vi "DriveControl.vi"(5 "RobotDriveDevRef":T1={"DevStatus"={"status"=FALSE, "code"=0, "source"=""}, "Motors[]"=[], "Square Inputs"=FALSE, "Max Output"=1.0, "Isochronous"=FALSE}, 7 "Xvalue of Target":dbl, 8 "Right axis value":dbl, 9 "Left axis value":dbl, 10 "Lower Bound":dbl, 11 "Upper Bound":dbl) -> ()   [LabVIEW 2011]
uses:
  <vilib>/Rock Robotics/WPI/RobotDrive/WPI_RobotDriveDevRef.ctl
  <vilib>/Rock Robotics/WPI/MotorControl/WPI_MotorControlDeviceRef.ctl
  <vilib>/Rock Robotics/SystemInterfaces/Typedef/FPGA_TypedefDigitalModule.ctl
  <vilib>/Rock Robotics/SystemInterfaces/DIO/FPGA_DIOPWMChannel.ctl
  <vilib>/Rock Robotics/WPI/PWM/WPI_PWMDeadband.ctl
  <vilib>/Rock Robotics/WPI/CAN/Jaguar/SubVIs/WPI_CANJaguar_ControlMode.ctl
  <vilib>/Rock Robotics/WPI/PWM/WPI_PWMTransform_ConPane.ctl
panel:
  in  "Joystick value":dbl
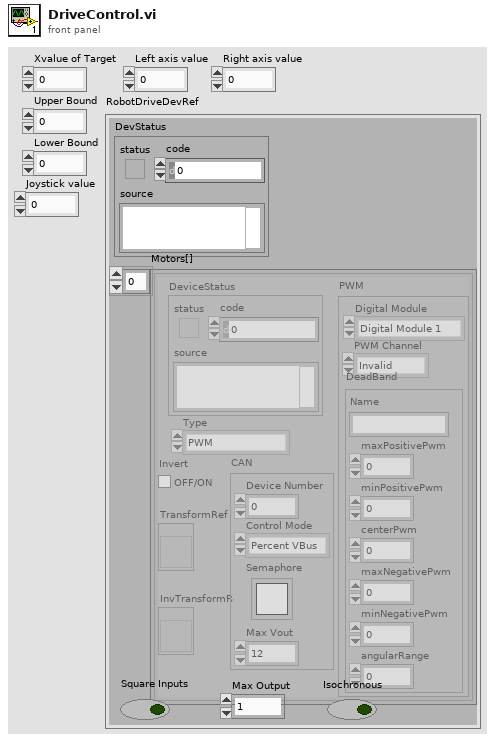
[diagram p1: front panel]
types:
  T1 = typedef "WPI_RobotDriveDevRef.ctl" = cluster{"DevStatus":errorcluster, "Motors[]":T2[], "Square Inputs":bool, "Max Output":dbl, "Isochronous":bool}
  T2 = typedef "WPI_MotorControlDeviceRef.ctl" = cluster{"DeviceStatus":errorcluster, "Type":enum16{"PWM", "CAN"}, "PWM":cluster{"Digital Module":T3, "PWM Channel":T4, "DeadBand":T5}, "CAN":cluster{"Device Number":u8, "Control Mode":T6, "Semaphore":T7, "Max Vout":dbl}, "Invert":bool, "TransformRef":T8, "InvTransformRef":T8}
  T3 = typedef "FPGA_TypedefDigitalModule.ctl" = enum16{"Digital Module 1", "Digital Module 2"}
  T4 = typedef "FPGA_DIOPWMChannel.ctl" = enum8{"PWM 1", "PWM 2", "PWM 3", "PWM 4", "PWM 5", "PWM 6", "PWM 7", "PWM 8", "PWM 9", "PWM 10", "Invalid"}
  T5 = typedef "WPI_PWMDeadband.ctl" = cluster{"Name":string, "maxPositivePwm":i32, "minPositivePwm":i32, "centerPwm":i32, "maxNegativePwm":i32, "minNegativePwm":i32, "angularRange":u16}
  T6 = typedef "WPI_CANJaguar_ControlMode.ctl" = enum8{"Percent VBus", "Current", "Speed", "Position", "Voltage"}
  T7 = typedef "Semaphore RefNum" = refnum<k1>
  T8 = typedef "WPI_PWMTransform_ConPane.ctl" = refnum<vi>
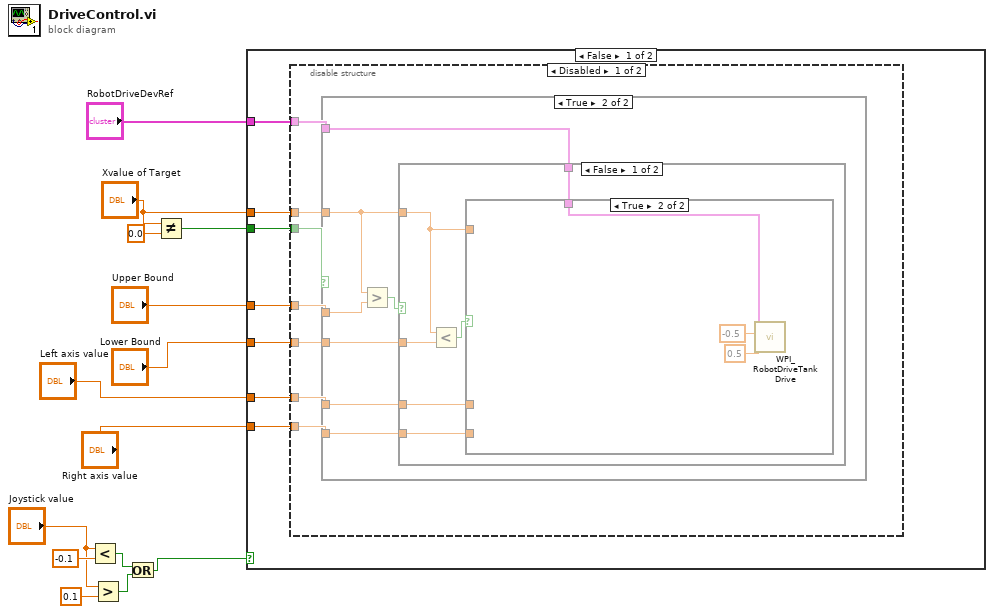
[diagram p0: block diagram]
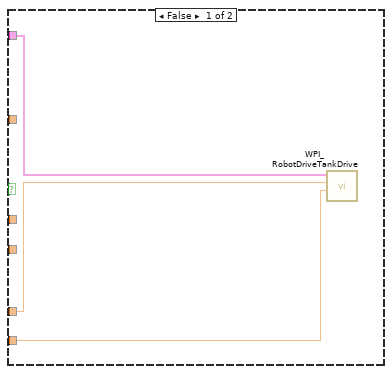
[diagram p2: hidden frame]
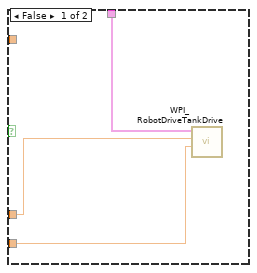
[diagram p3: hidden frame]
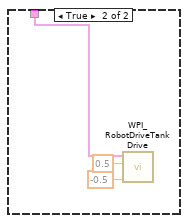
[diagram p4: hidden frame]
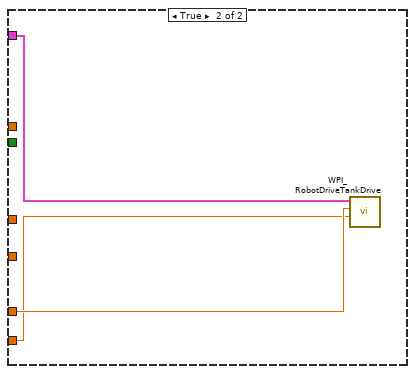
[diagram p6: hidden frame]
diagram:
  n1 = Less?(x="Joystick value", y=-0.1) -> (x < y?=w3:bool)
  n2 = Greater?(x="Joystick value", y=0.1) -> (0:w2:bool)
  n3 = Or(x=w3, y=w2) -> (x .or. y?=w1:bool)
  n4 = Not Equal?(x="Xvalue of Target", y=0.0) -> (x != y?=w13:bool)
  n5 = case shown="False" w1 {
    tunnel: w13 -> [w21 _]
    tunnel: "Xvalue of Target" -> [w20 _]
    tunnel: "Upper Bound" -> [w19 _]
    tunnel: "Lower Bound" -> [w18 _]
    tunnel: "RobotDriveDevRef" -> [w17 w56]
    tunnel: "Left axis value" -> [w16 w55]
    tunnel: "Right axis value" -> [w15 w54]
    frame False {
      n6 = disable-structure shown="Disabled" {
        disable-tunnel: w21 -> [w28 _]
        disable-tunnel: w20 -> [w27 _]
        disable-tunnel: w19 -> [w26 _]
        disable-tunnel: w18 -> [w25 _]
        disable-tunnel: w17 -> [w24 _]
        disable-tunnel: w16 -> [w23 _]
        disable-tunnel: w15 -> [w22 _]
        frame Disabled {
          n7 = case shown="True" w28 {
            tunnel: w27 -> [_ w36]
            tunnel: w26 -> [_ w38]
            tunnel: w25 -> [_ w35]
            tunnel: w24 -> [w31 w34]
            tunnel: w23 -> [w29 w33]
            tunnel: w22 -> [w30 w32]
            frame False {
              n8 = call <vilib>:"WPI_RobotDriveTankDrive.vi"("Right axis value"=w30, "Left axis value"=w29, "RobotDriveDevRef"=w31) -> ()  [unwired: 7 in, 2 out]
            }
            frame True {
              n9 = Greater?(x=w36, y=w38) -> (0:w37:bool)
              n10 = case shown="False" w37 {
                tunnel: w36 -> [w39 _]
                tunnel: w35 -> [w43 _]
                tunnel: w34 -> [w42 w53]
                tunnel: w33 -> [w41 _]
                tunnel: w32 -> [w40 _]
                frame False {
                  n11 = Less?(x=w39, y=w43) -> (x < y?=w44:bool)
                  n12 = case shown="True" w44 {
                    tunnel: w42 -> [w47 w50]
                    tunnel: w41 -> [w46 _]
                    tunnel: w40 -> [w45 _]
                    tunnel: w39 -> [_ _]
                    frame False {
                      n13 = call <vilib>:"WPI_RobotDriveTankDrive.vi"("Right axis value"=w45, "Left axis value"=w46, "RobotDriveDevRef"=w47) -> ()  [unwired: 7 in, 2 out]
                    }
                    frame True {
                      n14 = call <vilib>:"WPI_RobotDriveTankDrive.vi"("Right axis value"=0.5, "Left axis value"=-0.5, "RobotDriveDevRef"=w50) -> ()  [unwired: 7 in, 2 out]
                    }
                  }
                }
                frame True {
                  n15 = call <vilib>:"WPI_RobotDriveTankDrive.vi"("Right axis value"=-0.5, "Left axis value"=0.5, "RobotDriveDevRef"=w53) -> ()  [unwired: 7 in, 2 out]
                }
              }
            }
          }
        }
        frame Enabled {
        }
      }
    }
    frame True {
      n16 = call <vilib>:"WPI_RobotDriveTankDrive.vi"("Right axis value"=w54, "Left axis value"=w55, "RobotDriveDevRef"=w56) -> ()  [unwired: 7 in, 2 out]
    }
  }
